vi "AllThingsBaxter_ROS.vi"() -> ()   [LabVIEW 2012]
doc: "Collection of all ROS for LabVIEW VIs in the palette"
uses:
  <userlib>/ROS for LabVIEW Software/ROS/MessageBuilding/std_msgs/subs/boolScalar.vi
  <userlib>/ROS for LabVIEW Software/ROS/MessageBuilding/std_msgs/subs/durationScalar.vi
  <userlib>/ROS for LabVIEW Software/ROS/MessageBuilding/std_msgs/subs/float32Scalar.vi
  <userlib>/ROS for LabVIEW Software/ROS/MessageBuilding/std_msgs/subs/float64Scalar.vi
  <userlib>/ROS for LabVIEW Software/ROS/MessageBuilding/std_msgs/subs/i8Scalar.vi
  <userlib>/ROS for LabVIEW Software/ROS/MessageBuilding/std_msgs/subs/i16Scalar.vi
  <userlib>/ROS for LabVIEW Software/ROS/MessageBuilding/std_msgs/subs/i32Scalar.vi
  <userlib>/ROS for LabVIEW Software/ROS/MessageBuilding/std_msgs/subs/i64Scalar.vi
  <userlib>/ROS for LabVIEW Software/ROS/MessageBuilding/std_msgs/subs/stringScalar.vi
  <userlib>/ROS for LabVIEW Software/ROS/MessageBuilding/std_msgs/subs/timeScalar.vi
  <userlib>/ROS for LabVIEW Software/ROS/MessageBuilding/std_msgs/subs/u8Scalar.vi
  <userlib>/ROS for LabVIEW Software/ROS/MessageBuilding/std_msgs/subs/u16Scalar.vi
  <userlib>/ROS for LabVIEW Software/ROS/MessageBuilding/std_msgs/subs/u32Scalar.vi
  <userlib>/ROS for LabVIEW Software/ROS/MessageBuilding/std_msgs/subs/u64Scalar.vi
  <userlib>/ROS for LabVIEW Software/ROS/Code/_ROSDefinition.vi
  <userlib>/ROS for LabVIEW Software/ROS/MessageParsing/std_msgs/subs/parse_bool_scalar.vi
  <userlib>/ROS for LabVIEW Software/ROS/MessageParsing/std_msgs/subs/parse_duration_scalar.vi
  <userlib>/ROS for LabVIEW Software/ROS/MessageParsing/std_msgs/subs/parse_float32_scalar.vi
  <userlib>/ROS for LabVIEW Software/ROS/MessageParsing/std_msgs/subs/parse_float64_scalar.vi
  <userlib>/ROS for LabVIEW Software/ROS/MessageParsing/std_msgs/subs/parse_i16_scalar.vi
  <userlib>/ROS for LabVIEW Software/ROS/MessageParsing/std_msgs/subs/parse_i32_scalar.vi
  <userlib>/ROS for LabVIEW Software/ROS/MessageParsing/std_msgs/subs/parse_i64_scalar.vi
  <userlib>/ROS for LabVIEW Software/ROS/MessageParsing/std_msgs/subs/parse_i8_scalar.vi
  <userlib>/ROS for LabVIEW Software/ROS/MessageParsing/std_msgs/subs/parse_string_scalar.vi
  <userlib>/ROS for LabVIEW Software/ROS/MessageParsing/std_msgs/subs/parse_time_scalar.vi
  <userlib>/ROS for LabVIEW Software/ROS/MessageParsing/std_msgs/subs/parse_u16_scalar.vi
  <userlib>/ROS for LabVIEW Software/ROS/MessageParsing/std_msgs/subs/parse_u32_scalar.vi
  <userlib>/ROS for LabVIEW Software/ROS/MessageParsing/std_msgs/subs/parse_u64_scalar.vi
  <userlib>/ROS for LabVIEW Software/ROS/MessageParsing/std_msgs/subs/parse_u8_scalar.vi
  <userlib>/ROS for LabVIEW Software/ROS/MessageParsing/std_msgs/subs/parse_bool_array.vi
  <userlib>/ROS for LabVIEW Software/Devices/Baxter/BaxterVIs/LeftGripper.vi
  <userlib>/ROS for LabVIEW Software/Devices/Baxter/BaxterVIs/BothArmsPosition.vi
panel:
  out "ROS Master":string="192.168.1.110:11311"
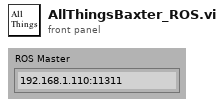
[diagram p1: front panel]
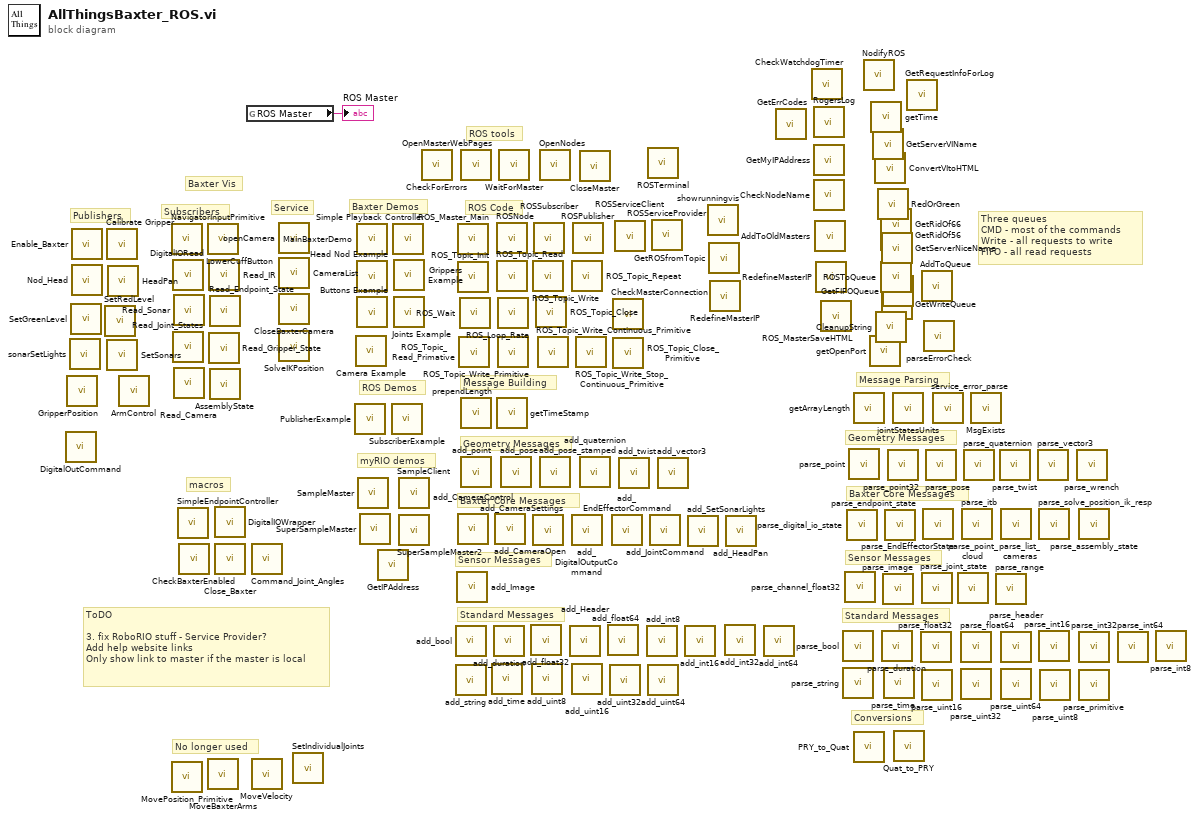
[diagram p0: block diagram]
diagram:
  # "No longer used"
  # "ToDO\n\n3. fix RoboRIO stuff - Service Provider?\nAdd help website links\nOnly show link to master if the master is local"
  # "Three queues\nCMD - most of the commands\nWrite - all requests to write\nFIFO - all read requests"
  # "Conversions"
  # "Standard Messages"
  # "Sensor Messages"
  # "Geometry Messages"
  # "Baxter Core Messages"
  # "Message Parsing"
  # "myRIO demos"
  # "ROS Demos"
  # "ROS tools"
  # "macros"
  # "Service"
  # "Subscribers"
  # "Publishers"
  # "Standard Messages"
  # "Sensor Messages"
  # "Baxter Core Messages"
  # "Geometry Messages"
  # "Message Building"
  # "ROS Code"
  # "Baxter Demos"
  # "Baxter Vis"
  n1 = call <userlib>:"DigitalOutCommand.vi"() -> ()  [unwired: 4 in, 1 out]
  n2 = call-poly <userlib>:"GripperPosition.vi"() -> ()  [unwired: 4 in, 1 out]
  n3 = call <userlib>:"sonarSetLights.vi"() -> ()  [unwired: 4 in, 1 out]
  n4 = call <userlib>:"SetGreenLevel.vi"() -> ()  [unwired: 4 in, 1 out]
  n5 = call <userlib>:"Enable_Baxter.vi"() -> ()  [unwired: 4 in, 1 out]
  n6 = call <userlib>:"Nod_Head.vi"() -> ()  [unwired: 4 in, 1 out]
  n7 = call <userlib>:"SetRedLevel.vi"() -> ()  [unwired: 4 in, 1 out]
  n8 = call <userlib>:"Calibrate Gripper.vi"() -> ()  [unwired: 4 in, 1 out]
  n9 = call <userlib>:"SetSonars.vi"() -> ()  [unwired: 4 in, 1 out]
  n10 = call <userlib>:"HeadPan.vi"() -> ()  [unwired: 4 in, 1 out]
  n11 = call-poly <userlib>:"ArmControl.vi"() -> ()  [unwired: 4 in, 1 out]
  n12 = call <userlib>:"NavigatorInputPrimitive.vi"() -> ()  [unwired: 3 in, 2 out]
  n13 = call <userlib>:"MovePosition_Primitive.vi"() -> ()  [unwired: 6 in, 1 out]
  n14 = call <userlib>:"DigitalIORead.vi"() -> ()  [unwired: 3 in, 2 out]
  n15 = call <userlib>:"Read_Joint_States.vi"() -> ()  [unwired: 3 in, 2 out]
  n16 = call <userlib>:"Read_Sonar.vi"() -> ()  [unwired: 3 in, 2 out]
  n17 = call <userlib>:"Read_Camera.vi"() -> ()  [unwired: 3 in, 2 out]
  n18 = call <userlib>:"SimpleEndpointController.vi"() -> ()  [unwired: 5 in, 1 out]
  n19 = call <userlib>:"CheckBaxterEnabled.vi"() -> ()  [unwired: 4 in, 1 out]
  n20 = call <userlib>:"LowerCuffButton.vi"() -> ()  [unwired: 3 in, 2 out]
  n21 = call <userlib>:"MoveBaxterArms.vi"() -> ()  [unwired: 6 in, 1 out]
  n22 = call <userlib>:"Read_IR.vi"() -> ()  [unwired: 3 in, 2 out]
  n23 = call <userlib>:"Read_Gripper_State.vi"() -> ()  [unwired: 3 in, 2 out]
  n24 = call <userlib>:"Read_Endpoint_State.vi"() -> ()  [unwired: 3 in, 2 out]
  n25 = call <userlib>:"AssemblyState.vi"() -> ()  [unwired: 3 in, 2 out]
  n26 = call <userlib>:"DigitalIOWrapper.vi"() -> ()  [unwired: 3 in, 2 out]
  n27 = call <userlib>:"Close_Baxter.vi"() -> ()  [unwired: 4 in, 1 out]
  n28 = global read "_ROSDefinition.vi" "ROS Master"() -> (→"ROS Master":string)
  n29 = call <userlib>:"Command_Joint_Angles.vi"() -> ()  [unwired: 6 in, 1 out]
  n30 = call <userlib>:"MoveVelocity.vi"() -> ()  [unwired: 6 in, 1 out]
  n31 = call <userlib>:"openCamera.vi"() -> ()  [unwired: 4 in, 1 out]
  n32 = call <userlib>:"CameraList.vi"() -> ()  [unwired: 3 in, 2 out]
  n33 = call <userlib>:"CloseBaxterCamera.vi"() -> ()  [unwired: 4 in, 1 out]
  n34 = call <userlib>:"SolveIKPosition.vi"() -> ()  [unwired: 3 in, 2 out]
  n35 = call <userlib>:"SetIndividualJoints.vi"() -> ()  [unwired: 6 in, 1 out]
  n36 = call <userlib>:"PublisherExample.vi"() -> ()  [unwired: 12 in]
  n37 = call <userlib>:"Camera Example.vi"() -> ()  [unwired: 12 in]
  n38 = call <userlib>:"MainBaxterDemo.vi"() -> ()  [unwired: 12 in]
  n39 = call <userlib>:"Head Nod Example.vi"() -> ()  [unwired: 12 in]
  n40 = call <userlib>:"Buttons Example.vi"() -> ()  [unwired: 12 in]
  n41 = call <userlib>:"SampleMaster.vi"() -> ()  [unwired: 12 in]
  n42 = call <userlib>:"SuperSampleMaster.vi"() -> ()  [unwired: 12 in]
  n43 = call <userlib>:"GetIPAddress.vi"() -> ()  [unwired: 3 in, 1 out]
  n44 = call <userlib>:"SubscriberExample.vi"() -> ()  [unwired: 12 in]
  n45 = call <userlib>:"Simple Playback Controller.vi"() -> ()  [unwired: 12 in]
  n46 = call <userlib>:"Grippers Example.vi"() -> ()  [unwired: 12 in]
  n47 = call <userlib>:"Joints Example.vi"() -> ()  [unwired: 12 in]
  n48 = call <userlib>:"SampleClient.vi"() -> ()  [unwired: 12 in]
  n49 = call <userlib>:"SuperSampleMaster2.vi"() -> ()  [unwired: 12 in]
  n50 = call <userlib>:"CheckForErrors.vi"() -> ()  [unwired: 2 in, 3 out]
  n51 = call-poly <userlib>:"add_bool.vi"() -> ()  [unwired: 5 in, 1 out]
  n52 = call-poly <userlib>:"add_string.vi"() -> ()  [unwired: 5 in, 1 out]
  n53 = call <userlib>:"add_Image.vi"() -> ()  [unwired: 5 in, 1 out]
  n54 = call <userlib>:"ROS_Master_Main.vi"() -> ()  [unwired: 4 in]
  n55 = call <userlib>:"ROS_Topic_Init.vi"() -> ()  [unwired: 3 in, 2 out]
  n56 = call <userlib>:"add_CameraControl.vi"() -> ()  [unwired: 5 in, 1 out]
  n57 = call <userlib>:"ROS_Topic_Read_Primative.vi"() -> ()  [unwired: 2 in, 3 out]
  n58 = call <userlib>:"ROS_Wait.vi"() -> ()  [unwired: 3 in, 2 out]
  n59 = call <userlib>:"OpenMasterWebPages.vi"() -> ()  [unwired: 4 in]
  n60 = call <userlib>:"prependLength.vi"() -> ()  [unwired: 5 in, 1 out]
  n61 = call <userlib>:"add_point.vi"() -> ()  [unwired: 5 in, 1 out]
  n62 = call-poly <userlib>:"add_time.vi"() -> ()  [unwired: 5 in, 1 out]
  n63 = call-poly <userlib>:"add_duration.vi"() -> ()  [unwired: 5 in, 1 out]
  n64 = call <userlib>:"add_CameraOpen.vi"() -> ()  [unwired: 5 in, 1 out]
  n65 = call <userlib>:"ROSNode.vi"() -> ()  [unwired: 4 in]
  n66 = call <userlib>:"ROS_Topic_Read.vi"() -> ()  [unwired: 3 in, 3 out]
  n67 = call <userlib>:"getTimeStamp.vi"() -> ()  [unwired: 2 in, 3 out]
  n68 = call <userlib>:"ROS_Loop_Rate.vi"() -> ()  [unwired: 5 in, 2 out]
  n69 = call <userlib>:"ROS_Topic_Write_Primitive.vi"() -> ()  [unwired: 3 in, 1 out]
  n70 = call <userlib>:"WaitForMaster.vi"() -> ()  [unwired: 1 in, 1 out]
  n71 = call <userlib>:"add_pose.vi"() -> ()  [unwired: 5 in, 1 out]
  n72 = call-poly <userlib>:"add_float32.vi"() -> ()  [unwired: 5 in, 1 out]
  n73 = call-poly <userlib>:"add_uint8.vi"() -> ()  [unwired: 5 in, 1 out]
  n74 = call <userlib>:"ROS_Topic_Write.vi"() -> ()  [unwired: 4 in, 2 out]
  n75 = call <userlib>:"add_CameraSettings.vi"() -> ()  [unwired: 5 in, 1 out]
  n76 = call <userlib>:"ROSSubscriber.vi"() -> ()  [unwired: 4 in]
  n77 = call <userlib>:"ROS_Topic_Close.vi"() -> ()  [unwired: 4 in, 1 out]
  n78 = call <userlib>:"ROS_Topic_Write_Continuous_Primitive.vi"() -> ()  [unwired: 3 in, 1 out]
  n79 = call <userlib>:"OpenNodes.vi"() -> ()  [unwired: 2 in]
  n80 = call <userlib>:"add_pose_stamped.vi"() -> ()  [unwired: 5 in, 1 out]
  n81 = call <userlib>:"add_Header.vi"() -> ()  [unwired: 5 in, 1 out]
  n82 = call <userlib>:"ROS_Topic_Repeat.vi"() -> ()  [unwired: 4 in, 2 out]
  n83 = call <userlib>:"add_DigitalOutputCommand.vi"() -> ()  [unwired: 5 in, 1 out]
  n84 = call-poly <userlib>:"add_uint16.vi"() -> ()  [unwired: 5 in, 1 out]
  n85 = call <userlib>:"ROSPublisher.vi"() -> ()  [unwired: 4 in]
  n86 = call <userlib>:"ROS_Topic_Write_Stop_Continuous_Primitive.vi"() -> ()  [unwired: 3 in, 1 out]
  n87 = call <userlib>:"CloseMaster.vi"() -> ()  [unwired: 3 in, 1 out]
  n88 = call <userlib>:"add_quaternion.vi"() -> ()  [unwired: 5 in, 1 out]
  n89 = call-poly <userlib>:"add_float64.vi"() -> ()  [unwired: 5 in, 1 out]
  n90 = call-poly <userlib>:"add_uint32.vi"() -> ()  [unwired: 5 in, 1 out]
  n91 = call <userlib>:"add_EndEffectorCommand.vi"() -> ()  [unwired: 5 in, 1 out]
  n92 = call <userlib>:"CheckMasterConnection.vi"() -> ()  [unwired: 2 in, 2 out]
  n93 = call <userlib>:"ROS_Topic_Close_Primitive.vi"() -> ()  [unwired: 3 in, 1 out]
  n94 = call <userlib>:"ROSServiceClient.vi"() -> ()  [unwired: 4 in]
  n95 = call <userlib>:"add_twist.vi"() -> ()  [unwired: 5 in, 1 out]
  n96 = call-poly <userlib>:"add_int8.vi"() -> ()  [unwired: 5 in, 1 out]
  n97 = call <userlib>:"ROSTerminal.vi"() -> ()  [unwired: 2 in]
  n98 = call-poly <userlib>:"add_uint64.vi"() -> ()  [unwired: 5 in, 1 out]
  n99 = call <userlib>:"add_JointCommand.vi"() -> ()  [unwired: 11 in, 1 out]
  n100 = call <userlib>:"ROSServiceProvider.vi"() -> ()  [unwired: 4 in]
  n101 = call <userlib>:"add_vector3.vi"() -> ()  [unwired: 5 in, 1 out]
  n102 = call-poly <userlib>:"add_int16.vi"() -> ()  [unwired: 5 in, 1 out]
  n103 = call <userlib>:"add_SetSonarLights.vi"() -> ()  [unwired: 5 in, 1 out]
  n104 = call <userlib>:"showrunningvis.vi"() -> ()  [unwired: 1 in]
  n105 = call <userlib>:"GetROSfromTopic.vi"() -> ()  [unwired: 2 in, 3 out]
  n106 = call <userlib>:"RedefineMasterIP.vi"() -> ()  [unwired: 2 in, 1 out]
  n107 = call-poly <userlib>:"add_int32.vi"() -> ()  [unwired: 5 in, 1 out]
  n108 = call <userlib>:"add_HeadPan.vi"() -> ()  [unwired: 11 in, 1 out]
  n109 = call-poly <userlib>:"add_int64.vi"() -> ()  [unwired: 5 in, 1 out]
  n110 = call <userlib>:"GetErrCodes.vi"() -> ()  [unwired: 2 in, 1 out]
  n111 = call <userlib>:"CheckWatchdogTimer.vi"() -> ()  [unwired: 6 in]
  n112 = call <userlib>:"RogersLog.vi"() -> ()  [unwired: 5 in, 2 out]
  n113 = call <userlib>:"GetMyIPAddress.vi"() -> ()  [unwired: 2 in, 2 out]
  n114 = call <userlib>:"CheckNodeName.vi"() -> ()  [unwired: 2 in, 2 out]
  n115 = call <userlib>:"AddToOldMasters.vi"() -> ()  [unwired: 4 in]
  n116 = call <userlib>:"RedefineMasterIP.vi"() -> ()  [unwired: 2 in, 1 out]
  n117 = call <userlib>:"ROS_MasterSaveHTML.vi"() -> ()  [unwired: 6 in]
  n118 = call-poly <userlib>:"parse_bool.vi"() -> ()  [unwired: 5 in, 3 out]
  n119 = call-poly <userlib>:"parse_string.vi"() -> ()  [unwired: 5 in, 3 out]
  n120 = call <userlib>:"parse_channel_float32.vi"() -> ()  [unwired: 5 in, 3 out]
  n121 = call <userlib>:"parse_digital_io_state.vi"() -> ()  [unwired: 5 in, 3 out]
  n122 = call <userlib>:"parse_point.vi"() -> ()  [unwired: 5 in, 3 out]
  n123 = call <userlib>:"getArrayLength.vi"() -> ()  [unwired: 5 in, 3 out]
  n124 = call <userlib>:"PRY_to_Quat.vi"() -> ()  [unwired: 2 in, 1 out]
  n125 = call <userlib>:"NodifyROS.vi"() -> ()  [unwired: 1 in, 1 out]
  n126 = call <userlib>:"getOpenPort.vi"() -> ()  [unwired: 1 out]
  n127 = call <userlib>:"getTime.vi"() -> ()  [unwired: 1 in, 1 out]
  n128 = call <userlib>:"GetServerVIName.vi"() -> ()  [unwired: 1 in, 1 out]
  n129 = call <userlib>:"ConvertVItoHTML.vi"() -> ()  [unwired: 1 in, 2 out]
  n130 = call <userlib>:"CleanupString.vi"() -> ()  [unwired: 1 in, 1 out]
  n131 = call <userlib>:"RedOrGreen.vi"() -> ()  [unwired: 1 in, 1 out]
  n132 = call <userlib>:"GetRidOf66.vi"() -> ()  [unwired: 1 in, 1 out]
  n133 = call <userlib>:"GetRidOf56.vi"() -> ()  [unwired: 1 in, 1 out]
  n134 = call <userlib>:"ROSToQueue.vi"() -> ()  [unwired: 4 in, 2 out]
  n135 = call <userlib>:"GetServerNiceName.vi"() -> ()  [unwired: 2 in, 1 out]
  n136 = call <userlib>:"GetWriteQueue.vi"() -> ()  [unwired: 4 in, 2 out]
  n137 = call-poly <userlib>:"parse_duration.vi"() -> ()  [unwired: 5 in, 3 out]
  n138 = call <userlib>:"GetFIFOQueue.vi"() -> ()  [unwired: 4 in, 2 out]
  n139 = call <userlib>:"parse_image.vi"() -> ()  [unwired: 4 in, 4 out]
  n140 = call-poly <userlib>:"parse_time.vi"() -> ()  [unwired: 5 in, 3 out]
  n141 = call <userlib>:"parse_endpoint_state.vi"() -> ()  [unwired: 5 in, 3 out]
  n142 = call <userlib>:"parse_point32.vi"() -> ()  [unwired: 5 in, 3 out]
  n143 = call <userlib>:"jointStatesUnits.vi"() -> ()  [unwired: 3 in, 3 out]
  n144 = call <userlib>:"Quat_to_PRY.vi"() -> ()  [unwired: 2 in, 1 out]
  n145 = call <userlib>:"GetRequestInfoForLog.vi"() -> ()  [unwired: 1 in, 1 out]
  n146 = call-poly <userlib>:"parse_float32.vi"() -> ()  [unwired: 5 in, 3 out]
  n147 = call <userlib>:"AddToQueue.vi"() -> ()  [unwired: 5 in, 1 out]
  n148 = call <userlib>:"parse_joint_state.vi"() -> ()  [unwired: 4 in, 4 out]
  n149 = call-poly <userlib>:"parse_uint16.vi"() -> ()  [unwired: 5 in, 3 out]
  n150 = call <userlib>:"parse_EndEffectorState.vi"() -> ()  [unwired: 5 in, 3 out]
  n151 = call <userlib>:"parseErrorCheck.vi"() -> ()  [unwired: 3 in, 1 out]
  n152 = call <userlib>:"parse_pose.vi"() -> ()  [unwired: 5 in, 3 out]
  n153 = call <userlib>:"service_error_parse.vi"() -> ()  [unwired: 3 in, 3 out]
  n154 = call <userlib>:"parse_point_cloud.vi"() -> ()  [unwired: 4 in, 4 out]
  n155 = call-poly <userlib>:"parse_float64.vi"() -> ()  [unwired: 5 in, 3 out]
  n156 = call-poly <userlib>:"parse_uint32.vi"() -> ()  [unwired: 5 in, 3 out]
  n157 = call <userlib>:"parse_itb.vi"() -> ()  [unwired: 5 in, 3 out]
  n158 = call <userlib>:"parse_quaternion.vi"() -> ()  [unwired: 5 in, 3 out]
  n159 = call <userlib>:"MsgExists.vi"() -> ()  [unwired: 10 in, 2 out]
  n160 = call <userlib>:"parse_range.vi"() -> ()  [unwired: 4 in, 4 out]
  n161 = call <userlib>:"parse_twist.vi"() -> ()  [unwired: 5 in, 3 out]
  n162 = call <userlib>:"parse_list_cameras.vi"() -> ()  [unwired: 5 in, 3 out]
  n163 = call <userlib>:"parse_header.vi"() -> ()  [unwired: 5 in, 3 out]
  n164 = call-poly <userlib>:"parse_uint64.vi"() -> ()  [unwired: 5 in, 3 out]
  n165 = call <userlib>:"parse_vector3.vi"() -> ()  [unwired: 5 in, 3 out]
  n166 = call <userlib>:"parse_solve_position_ik_resp.vi"() -> ()  [unwired: 4 in, 4 out]
  n167 = call-poly <userlib>:"parse_int16.vi"() -> ()  [unwired: 5 in, 3 out]
  n168 = call-poly <userlib>:"parse_uint8.vi"() -> ()  [unwired: 5 in, 3 out]
  n169 = call <userlib>:"parse_wrench.vi"() -> ()  [unwired: 5 in, 3 out]
  n170 = call <userlib>:"parse_assembly_state.vi"() -> ()  [unwired: 3 in, 4 out]
  n171 = call-poly <userlib>:"parse_int32.vi"() -> ()  [unwired: 5 in, 3 out]
  n172 = call-poly <userlib>:"parse_primitive.vi"() -> ()  [unwired: 5 in, 3 out]
  n173 = call-poly <userlib>:"parse_int64.vi"() -> ()  [unwired: 5 in, 3 out]
  n174 = call-poly <userlib>:"parse_int8.vi"() -> ()  [unwired: 5 in, 3 out]
